vi "DFSIterator_Init.vi"(0 "object in":refnum<class "DFSTreeIterator.lvclass">, 2 "ItearableCollection":refnum<class "Tree.lvclass">, 5 "Error In":errorcluster) -> (14 "object out":refnum<class "DFSTreeIterator.lvclass">, 19 "Error Out":errorcluster)   [LabVIEW 2024, in "DFSTreeIterator.lvclass"]
uses:
  DFSTreeIterator.lvclass
  Tree_class/Tree.lvclass
  Support/Stack_class/Stack.lvclass
  DFSTreeIterator.lvclass/DFSTreeIterator.ctl
  Node_class/Node.lvclass
panel:
  # "Connector Pane"
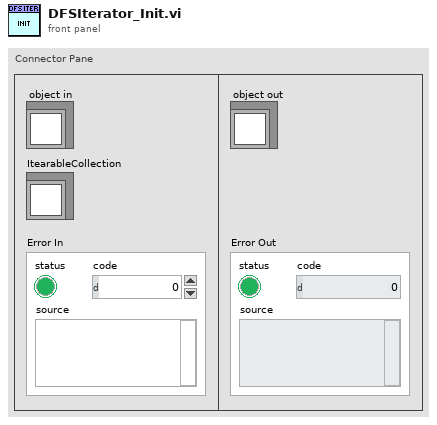
[diagram p1: front panel]
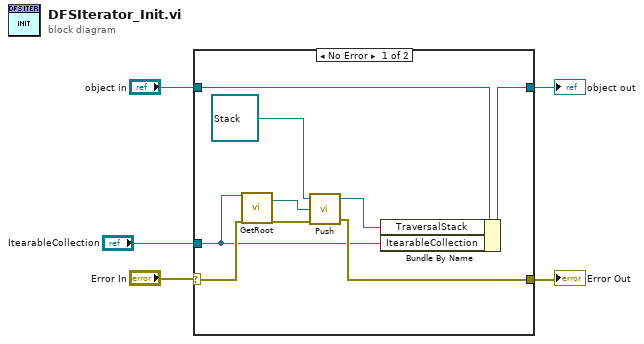
[diagram p0: block diagram]
diagram:
  n1 = case shown="No Error" "Error In" {
    selector: "Error In" -> [w9 w15]
    tunnel: "object in" -> [w14 w16]
    tunnel: [w13 w16] -> w4
    tunnel: [w11 w15] -> w2
    tunnel: "ItearableCollection" -> [w8 _]
    frame No Error {
      n2 = call-dynamic "GetRoot.vi"("object in"=w8, "Error In"=w9) -> ("Root"=w7:refnum<class "Node.lvclass">, "Error Out"=w10:errorcluster)  [unwired: 15 in, 1 out]
      n3 = call-dynamic "Push.vi"("Error In"=w10, "Data"=w7, "object in"=refnum<class "Stack.lvclass"> refnum ("Stack")) -> ("Error Out"=w11:errorcluster, "object out"=w6:refnum<class "Stack.lvclass">)  [unwired: 1 in]
      n4 = Bundle By Name(cluster=w14, "TraversalStack"=w6, "ItearableCollection"=w8) -> (w13:refnum<class "DFSTreeIterator.lvclass">)
    }
    frame Error {
    }
  }
  "object out" <- w4
  "Error Out" <- w2
